vi "PassFail.vi"(11 "Pass?":bool) -> (3 "Result":string)   [LabVIEW 2015, in "Test Actuator State.lvclass"]
uses:
  States/Test Actuator State/Test Actuator State.lvclass
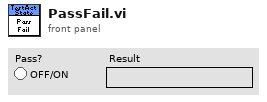
[diagram p1: front panel]
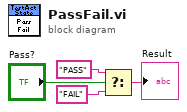
[diagram p0: block diagram]
diagram:
  n1 = Select(t="PASS", s="Pass?", f="FAIL") -> (s? t:f=→"Result":string)
